vi "Write TestCaseMap.vi"(10 "TestCaseMap":map{string, set{string}}(c390), 11 "RequirementsFile in":refnum<class "TraceabilityMatrix.lvclass">) -> (3 "RequirementsFile out":refnum<class "TraceabilityMatrix.lvclass">)   [LabVIEW 2021, in "Bananas.lvlib" / "TraceabilityMatrix.lvclass"]
uses:
  TraceabilityMatrix.lvclass
  TraceabilityMatrix.lvclass/TraceabilityMatrix.ctl
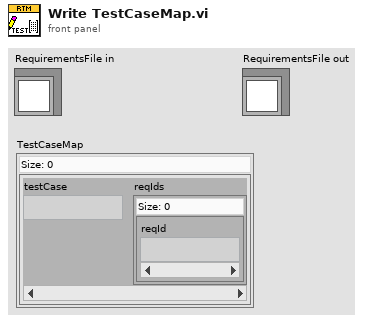
[diagram p1: front panel]
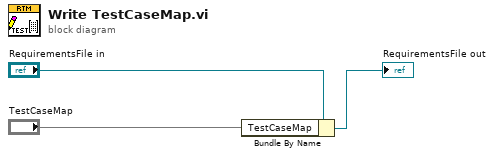
[diagram p0: block diagram]
diagram:
  n1 = Bundle By Name(cluster="RequirementsFile in", "TestCaseMap"="TestCaseMap") -> (→"RequirementsFile out":refnum<class "TraceabilityMatrix.lvclass">)
